vi "SetMotorType.vi"(8 "error in":errorcluster, 10 "Type":i32, 11 "PicomotorController in":refnum<class "PicomotorController.lvclass">) -> (0 "error out":errorcluster, 3 "PicomotorController out":refnum<class "PicomotorController.lvclass">)   [LabVIEW 2020, in "PicomotorController.lvclass"]
uses:
  PicomotorController.lvclass
  MCL Cmd Cluster.ctl
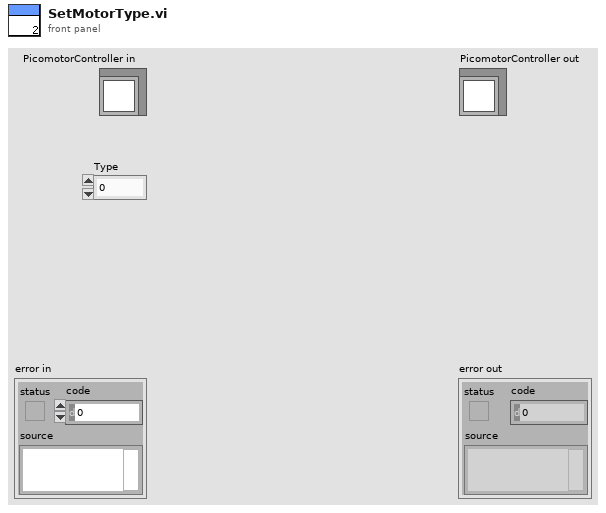
[diagram p1: front panel]
types:
  T1 = typedef "MCL Cmd Cluster.ctl" = cluster{"MCL Cmd":enum16{"User....", "DEF", "DIAG", "INI", "LOCK", "UNLOCK", "MAP", "SAV", "VER", "ACC", "CHL", "FOR", "GO", "HAL", "MOF", "MON", "MPV", "POS", "REL", "REV", "STA", "STO", "TYP", "VEL", "ABS", "SER", "NOS", "DRT", "FLI", "RLI", "FIN", "RIN", "AIN", "IN", "JOF", "JON", "OUT", "RES FINE", "RES COARSE", "02 (HEX)", "PWM", "CNT", "TMR", "HOSTNAME", "IPADDR", "IPMODE", "NETMASK", "GATEWAY", "DNSSRVR", "PASSWD", "ECHO", "MACADDR"}, "User Cmd/Numeric Argu":string, "Query/Set":enum16{"Query", "Set"}}
  T2 = typedef "VISA & TCPIP Control.ctl" = cluster{"Resource Name":refnum<visa-resource-name>, "Init VISA":bool, "Close VISA":bool, "VISA or TCP/IP":bool, "IP Address/Hostname":string}
  T3 = typedef "Pico Parameters.ctl" = cluster{"Pico Type":enum16{"Open-Loop Pico", "Close-Loop Pico", "Pico Ultra"}, "Acceleration (steps/sec^2)":string, "Velocity ( Hz)":string, "Driver":string, "Motor":string, "Channel":string, "Process Step":string}
  T4 = typedef "Error.ctl" = errorcluster
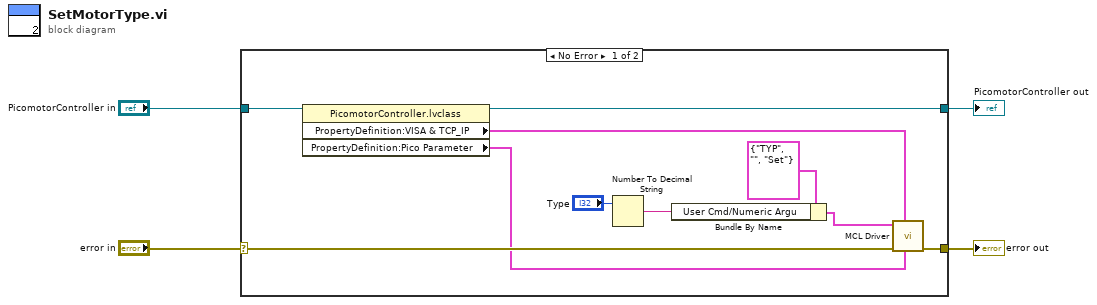
[diagram p0: block diagram]
diagram:
  n1 = case shown="No Error" "error in" {
    selector: "error in" -> [w10 w16]
    tunnel: [w9 w16] -> w3
    tunnel: [w11 w15] -> w1
    tunnel: "PicomotorController in" -> [w12 w15]
    frame No Error {
      n2 = property class="PicomotorController.lvclass"(reference=w12) -> (reference out=w11:refnum<class "PicomotorController.lvclass">, "PropertyDefinition:VISA & TCP_IP"=w14:T2, "PropertyDefinition:Pico Parameter"=w8:T3)  [unwired: 1 in, 1 out]
      n3 = Number To Decimal String(number="Type") -> (decimal integer string=w6:string)  [unwired: 1 in]
      n4 = Bundle By Name(cluster=T1 {"MCL Cmd"=enum."TYP", "User Cmd/Numeric Argu"="", "Query/Set"=enum."Set"} ("MCL Command"), "User Cmd/Numeric Argu"=w6) -> (w7:T1)
      n5 = call "MCL Driver.vi"("Pico Parameter"=w8, "VISA"=w14, "Error In (no error)"=w10, "MCL Command"=w7) -> ("Error Out"=w9:T4)  [unwired: 3 in, 4 out]
    }
    frame Error {
    }
  }
  "error out" <- w3
  "PicomotorController out" <- w1
